vi "mainVI.vi"() -> ()   [LabVIEW 2019]
uses:
  <vilib>/Platform/TimedLoop/XDataNode/timing_clust.ctl
  <vilib>/Platform/TimedLoop/XDataNode/nitl_modes.ctl
  <vilib>/Platform/TimedLoop/XDataNode/wakeup.ctl
  <extravilib>/ChannelInstances/Tag-bool/Read With Abort.vi
  <extravilib>/ChannelInstances/Tag-bool/Write With Abort.vi
  <extravilib>/ChannelInstances/Tag-bool/Instantiate.vi
  <extravilib>/ChannelInstances/Tag-bool/EndpointRead.vi
  <extravilib>/ChannelInstances/Tag-bool/Endpoint.vi
  <vilib>/Platform/TimedLoop/XDataNode/XDataNode.xnode
  <vilib>/Platform/TimedLoop/XDataNode/XDNodeRunTimeDep.lvlib
  <extravilib>/ChannelInstances/Tag-bool.lvlib
  <instrlib>/Sefram DAS240/Sefram DAS240.lvlib
panel:
  out "Numéro de la prochaine analyse":i32
  in  "Periode d'échantillonage":u16(ring)=6 items=["1 Millisecond", "2 Milliseconds", "5 Milliseconds", "10 Milliseconds", "20 Milliseconds", "50 Milliseconds", "100 Milliseconds", "200 Milliseconds", "500 Milliseconds", "1 Second", "2 Seconds", "5 Seconds", "10 Seconds", "20 Seconds", "1 Minute", "2 Minutes", "5 Minutes", "10 Minutes", "20 Minutes"]
  in  "Nom VISA DAS240":refnum<visa-resource-name>="DAS240"
  in  "Generer nouveau":bool
  in  "Chemin de sortie":path=path "C:/Users/manip/Documents/Thermo aquisition data/labview/output"
  out "Haute temperature":bool
  in  "Température maximale":dbl=100.0 caption="Fréequence d'échantillonage (Hz)"
  in  "Nom de l'analyse":string="sys1_isoPla"
  out "Prêt":bool
  in  "START":bool
  in  "stop":bool
  out "Signal de sortie":dbl(graph)
  out "Signal d'entrée mesuré":cluster{"Numeric":dbl, "Numeric":dbl}(graph)
  out "Das trouvé":bool
  out "Signal d'entrée":cluster{dbl[], dbl[]}(graph)
  out "DSP par FFT":cluster{dbl[], dbl[]}(graph)
  out "Alim connectée":bool
  in  "Fréequence \nd'échantillonage (alim)":dbl=1.0 caption="Fréequence d'échantillonage (Hz)"
  in  "Numéro de la machine voulu":string="2196400002"
  in  "Generation de données":enum32{"Labview", "CSV"}(tab)
  in  "Labview opt":T1={"Fréequence maximale (Hz)"=0.1, "Temps de simulation (min)"=2.0, "Amplitude minimale (V)"=0.0, "Amplitude maximale (V)"=1.0}
  in  "Chemin du fichier":path=path "C:/Users/manip/Documents/Thermo aquisition data/labview/input/data.csv"
  out "Machines trouvées":string[][](array[string])=[["COM7", "PSI 9200-25", "2196400002", "06230310", "", "200,0000", "25,0000", "1500,0000", "0,0000", "240,0000", "33", "PSI 9000 Series", "0", "", "", "", "", "V2.31 24.08.2020", "V2.20 20.11.2020", "V1.6.6", "Modbus_RTU"], ["TCPIP0::169.254.133.212::502::SOCKET", "", "", "", "///", "0,000", "0,000", "0,000", "", "", "0", "Ethernet", "0", "", "", "", "", "", "", "", "Can"]]
  out "Sortie d'erreur":errorcluster
  # "Génération des données"
  # "Acquisition des données"
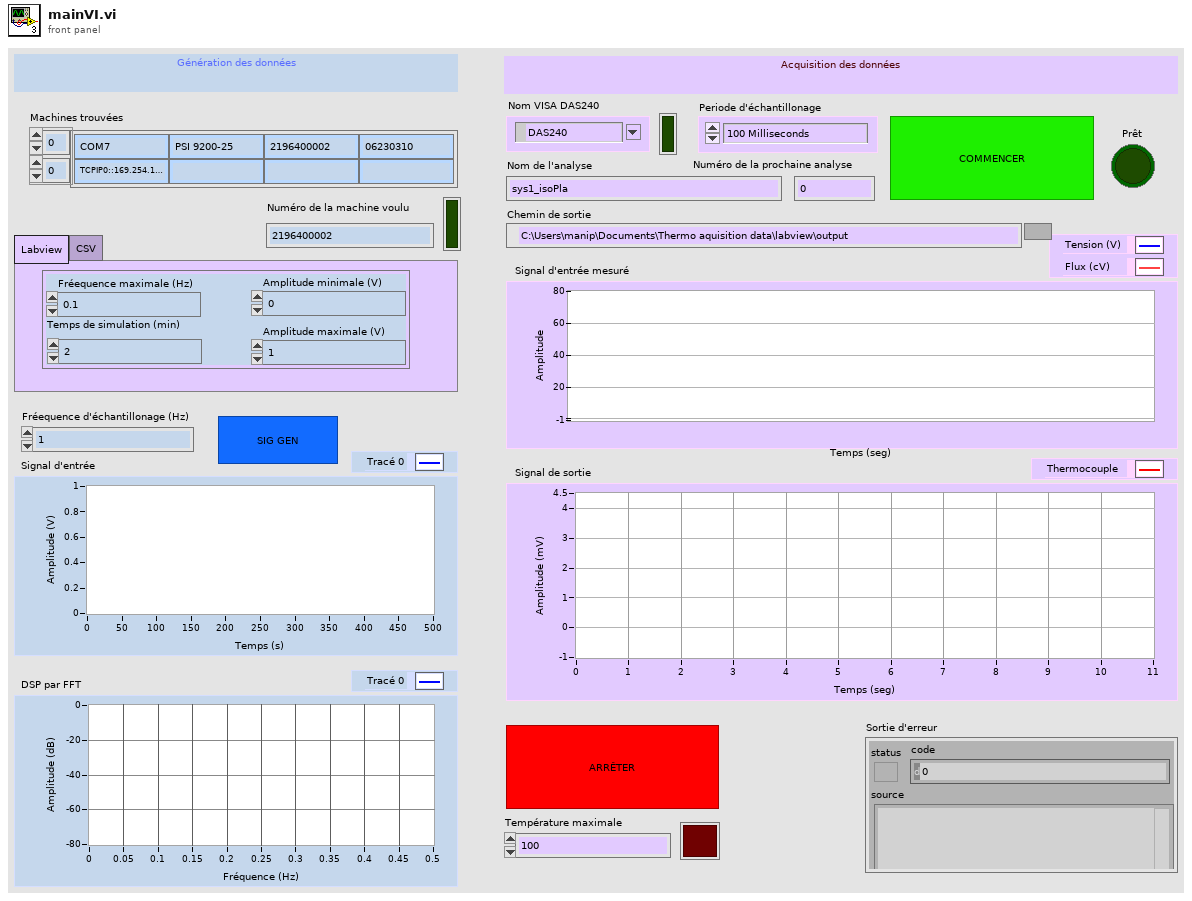
[diagram p1: front panel]
types:
  T1 = cluster{"Fréequence maximale (Hz)":dbl, "Temps de simulation (min)":dbl, "Amplitude minimale (V)":dbl, "Amplitude maximale (V)":dbl}
  T2 = cluster{"Device information out":string[], "VISA resource name out":refnum<visa-resource-name>, "refnum en sortie":refnum<file>}
  T3 = typedef "XDNodeRunTimeDep.lvlib/timing_clust.ctl" = cluster{"Expected End [f-1]":u64, "Actual End [f-1]":u64, "Finished Late? [f-1]":bool, "Expected End [i-1]":u64, "Actual End [i-1]":u64, "Finished Late? [i-1]":bool, "Expected Start [i]":u64, "Actual Start [i]":u64, "Expected Start [f]":u64, "Actual Start [f]":u64, "Source Name":string, "Structure Name":string, "Period":i64, "Deadline":i64, "Offset":i64, "Start":i64, "Priority":i32, "Timeout":i32, "Mode":T4, "Wakeup Reason":T5, "Error":errorcluster, "Source Type":string, "Secondary Source Type":string, "Global End Time":u64, "Global Start Time":u64, "Frame Duration":u64, "Iteration Duration":u64, "Assigned CPU":i32, "I/O Scan Engine Mode":u32}
  T4 = typedef "XDNodeRunTimeDep.lvlib/nitl_modes.ctl" = enum32{"No Change", "Process missed periods, maintain original phase", "Discard missed periods, maintain original phase", "Process missed periods, ignore original phase", "Discard missed periods, ignore original phase"}
  T5 = typedef "XDNodeRunTimeDep.lvlib/wakeup.ctl" = enum32{"Normal", "Aborted", "Asynchronous wakeup", "Timing source error", "Timed loop error", "Timeout"}
  T6 = typedef "Tag-bool.lvlib/))Channel.ctl" = refnum<queue>
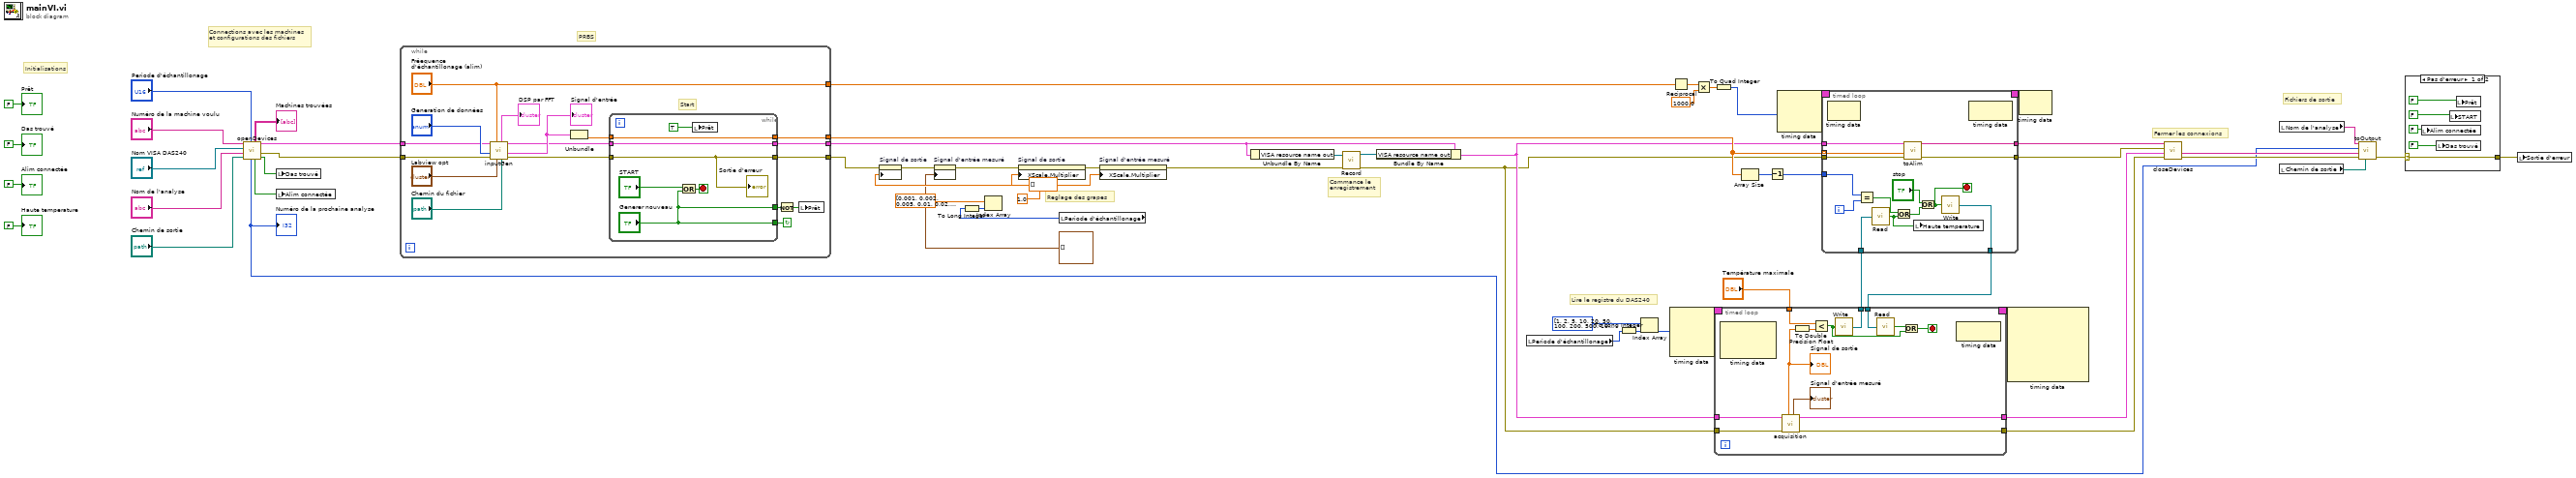
[diagram p0: block diagram]
diagram:
  w10 = 1.0 ("Échelle des X.Offset et multiplicateur:Multiplicateur")
  # "Fichiers de sortie"
  # "Commance le\nenregistrement"
  # "PRBS"
  # "Initialisations"
  # "Reglage des grapes"
  # "Fermer les connexions"
  # "Lire le registre du DAS240"
  # "Connections avec les machines\net configurations des fichiers"
  n1 = call "openDevices.vi"("Record Period"="Periode d'échantillonage", "Chemin de sortie"="Chemin de sortie", "Nom de l'analyse"="Nom de l'analyse", "Nom VISA d'entrée"="Nom VISA DAS240", "Numéro de série (PSI - 9200)"="Numéro de la machine voulu") -> ("Das trouvé/configuré"=w15:bool, "Erreur de sortie"=w16:errorcluster, "ID de sortie"=w35:T2, "Alim connectée"=w14:bool, "Machines trouvées"=→"Machines trouvées":string[][], "Numéro de la\nprochaine analyse"=w1:i32)  [unwired: 1 in]
  "Numéro de la prochaine analyse" <- w1
  n2 = local write "Das trouvé"(w15) -> ()
  n3 = local write "Alim connectée"(w14) -> ()
  n4 = while {
    tunnel: ["Fréequence \nd'échantillonage (alim)"] -> w50
    tunnel: [w69] -> w47
    tunnel: w16 -> [w68]
    tunnel: w35 -> [w67]
    tunnel: [w61] -> w28
    tunnel: [w66] -> w9
    stop <- w64 continue-if-true
    # "Start"
    n5 = call "inputGen.vi"("Chemin du fichier"="Chemin du fichier", "Labview opt"="Labview opt", "Fréequence \nd'échantillonage (alim)"="Fréequence \nd'échantillonage (alim)", "Entrée d'erreur"=w68, "Commande onglets"="Generation de données", "ID d'entrée"=w67) -> ("Sortie d'erreur"=w65:errorcluster, "Signal d'entrée"=w72:cluster{dbl[], dbl[]}, "ID de sortie"=w71:T2, "DSP par FFT"=→"DSP par FFT":cluster{dbl[], dbl[]})  [unwired: 2 in]
    "Signal d'entrée" <- w72
    n6 = Unbundle(w72) -> (w70:dbl[])  [unwired: 1 out]
    n7 = while {
      tunnel: w71 -> [w84]
      tunnel: [w84] -> w66
      tunnel: [w83] -> w69
      tunnel: w70 -> [w83]
      tunnel: [w82] -> w61
      tunnel: w65 -> [w82]
      tunnel: ["Generer nouveau"] -> w64
      tunnel: ["Generer nouveau"] -> w63
      stop <- w80 stop-if-true
      n8 = Or(x="START", y="Generer nouveau") -> (x .or. y?=w80:bool)
      n9 = local write "Prêt"(TRUE ("START")) -> ()
      "Sortie d'erreur" <- w82
    }
    n10 = Not(x=w63) -> (.not. x?=w62:bool)
    n11 = local write "Prêt"(w62) -> ()
  }
  n12 = property on="Signal de sortie" class="GraphDér (strict)"(error in=w28, "History Data"=sgl[] [] ("Données d'historique")) -> (error out=w37:errorcluster)  [unwired: 1 in, 1 out]
  n13 = property on="Signal d'entrée mesuré" class="GraphDér (strict)"(error in=w37, "History Data"=cluster{"Numeric":dbl, "Numeric":dbl}[] [] ("Données d'historique")) -> (error out=w36:errorcluster)  [unwired: 1 in, 1 out]
  n14 = property on="Signal de sortie" class="GraphDér (strict)"(error in=w36, "XScale.Multiplier"=w10) -> (error out=w29:errorcluster)  [unwired: 1 in, 1 out]
  n15 = local read "Periode d'échantillonage"() -> (w24:u16)
  n16 = To Long Integer(number=w24) -> (32bit integer=w25:i32)
  n17 = Index Array(array=dbl[] [0.001, 0.002, 0.005, 0.01, 0.02, 0.05, 0.1, 0.2, 0.5, 1.0, 2.0, 5.0, 10.0, 20.0, 60.0, 120.0, 300.0], index=w25) -> ()  [unwired: 1 out]
  n18 = property on="Signal d'entrée mesuré" class="GraphDér (strict)"(error in=w29, "XScale.Multiplier"=w10) -> (error out=w27:errorcluster)  [unwired: 1 in, 1 out]
  n19 = Unbundle By Name(w9) -> ("VISA resource name out"=w8:refnum<visa-resource-name>)
  n20 = call <instrlib>:"Record.vi"("error in (no error)"=w27, "VISA resource name"=w8) -> ("error out"=w3:errorcluster, "VISA resource name out"=w7:refnum<visa-resource-name>)  [unwired: 8 in]
  n21 = Bundle By Name(cluster=w9, "VISA resource name out"=w7) -> (w6:T2)
  n22 = local read "Periode d'échantillonage"() -> (w21:u16)
  n23 = To Long Integer(number=w21) -> (32bit integer=w22:i32)
  n24 = Index Array(array=i64[] [1, 2, 5, 10, 20, 50, 100, 200, 500, 1000, 2000, 5000, 10000, 20000, 60000, 120000, 300000], index=w22) -> (element=w20:i64)
  n25 = node-c288(w20) -> (w55:T3)  [unwired: 3 in]
  n26 = Reciprocal(x=w50) -> (1/x=w41:dbl)
  n27 = Multiply(x=w41, y=1000.0) -> (x*y=w57:dbl)
  n28 = To Quad Integer(1:w57) -> (0:w56:i64)
  n29 = Array Size(array=w47) -> (size(s)=w46:i32)
  n30 = Decrement(x=w46) -> (x-1=w45:i32)
  n31 = node-c288(w56) -> (w60:T3)  [unwired: 2 in]
  n32 = local read "Nom de l'analyse"() -> (w19:string)
  n33 = local read "Chemin de sortie"() -> (w13:path)
  n34 = timed-loop {
    timing: w55 -> [_]
    timing-out: [_] -> w54
    tunnel: w6 -> [w90]
    tunnel: w3 -> [w89]
    tunnel: w49 -> [w97]
    tunnel: [w96] -> w44
    tunnel: "Température maximale" -> [w92]
    tunnel: [w86] -> w5
    tunnel: [w85] -> w4
    stop <- w93 stop-if-true
    n35 = node-c288() -> ()  [unwired: 1 in, 3 out]
    n36 = call "acquisition.vi"("Erreur en entrée"=w89, "ID d'entrée"=w90) -> ("sortie d'erreur"=w86:errorcluster, "ID de sortie"=w85:T2, "Graphe de l'entrée"=→"Signal d'entrée mesuré":cluster{"Numeric":dbl, dbl}, "Graph de la sortie"=w88:dbl)  [unwired: 6 in]
    "Signal de sortie" <- w88
    n37 = To Double Precision Float(number=w88) -> (double precision float=w91:dbl)
    n38 = Less?(x=w92, y=w91) -> (x < y?=w94:bool)
    n39 = call <extravilib>:"Write.vi"("element"=w94) -> ("channel"=w96:T6)  [unwired: 1 out]
    n40 = call <extravilib>:"Read.vi"("channel"=w97) -> ("element"=w95:bool)  [unwired: 1 in, 1 out]
    n41 = Or(x=w95, y=w94) -> (x .or. y?=w93:bool)
    n42 = node-c288() -> ()  [unwired: 1 in, 1 out]
  }
  n43 = timed-loop {
    timing: w60 -> [_]
    timing-out: [_] -> w59
    tunnel: w6 -> [w104]
    tunnel: w3 -> [w102]
    tunnel: [w100] -> w51
    tunnel: [w101] -> w52
    tunnel: w47 -> [w103] mode=indexing
    tunnel: [w113] -> w49
    tunnel: w45 -> [w112]
    tunnel: w44 -> [w106]
    i -> [w111]
    stop <- w110 stop-if-true
    n44 = node-c288() -> ()  [unwired: 1 in, 1 out]
    n45 = Equal?(x=w112, y=w111) -> (x = y?=w107:bool)
    n46 = call <extravilib>:"Read.vi"("channel"=w106) -> ("element"=w105:bool)  [unwired: 1 in, 1 out]
    n47 = Or(x=w107, y=w105) -> (x .or. y?=w108:bool)
    n48 = call "toAlim.vi"("Error in"=w102, "Entree"=w103, "ID d'entrée"=w104) -> ("Erreur en sortie"=w100:errorcluster, "Device information out"=w101:string[])  [unwired: 7 in]
    n49 = local write "Haute temperature"(w105) -> ()
    n50 = Or(x="stop", y=w108) -> (x .or. y?=w110:bool)
    n51 = call <extravilib>:"Write.vi"("element"=w110) -> ("channel"=w113:T6)  [unwired: 1 out]
    n52 = node-c288() -> ()  [unwired: 1 in, 1 out]
  }
  n53 = node-c288(w54) -> ()  [unwired: 7 out]
  n54 = node-c288(w59) -> ()  [unwired: 1 out]
  n55 = call "closeDevices.vi"("Erreur d'entrée DAS"=w5, "ID a l'entrée"=w4, "Erreur d'entrée alim"=w51, "Device information in"=w52) -> ("Erreur de sortie"=w18:errorcluster, "TCP/IP Settings:Dot-Notation Address"=w2:string)  [unwired: 6 in]
  n56 = call "toOutput.vi"("Chemin de sortie"=w13, "Erreur en entrée"=w18, "IP DAS240"=w2, "Num de l'analyse"=w1, "Nom de l'analyse"=w19) -> ("Erreur en sortie"=w17:errorcluster)  [unwired: 6 in]
  n57 = case shown="Pas d'erreur" w17 {
    selector: w17 -> [w120 w121]
    tunnel: [w120 w121] -> w12
    frame No Error {
      n58 = local write "Alim connectée"(FALSE ("element")) -> ()
      n59 = local write "Das trouvé"(FALSE ("element")) -> ()
      n60 = local write "START"(FALSE ("element")) -> ()
      n61 = local write "Prêt"(FALSE ("element")) -> ()
    }
    frame Error {
    }
  }
  n62 = local write "Sortie d'erreur"(w12) -> ()
  "Alim connectée" <- FALSE ("Alim connectée")
  "Das trouvé" <- FALSE ("Das trouvé")
  "Prêt" <- FALSE ("Ready")
  "Haute temperature" <- FALSE ("Haute temperature")
